vi "ConfigToIni.vi"(8 "Error In":errorcluster[](array[cluster]), 11 "ConfigRef":refnum<class "Config.lvclass">) -> (0 "Error Out":errorcluster[](array[cluster]), 3 "ConfigRef":refnum<class "Config.lvclass">)   [LabVIEW 2014, in "Config_class.lvlib" / "Config.lvclass"]
uses:
  Config.lvclass
  Typedefs/eLogLvl.ctl
  Config.lvclass/Config.ctl
  Accessors/Read ConfigFilePath.vi
  Accessors/Read Logging.vi
  Accessors/Read Root Directory.vi
  <vilib>/Utility/config.llb/NI_LVConfig.lvlib
  <userlib>/NIST/NISTErrorLib/NISTErrorLib.lvlib
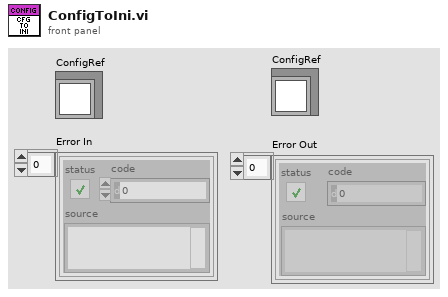
[diagram p1: front panel]
types:
  T1 = cluster{"pathRootDir":path, "OutDir":string, "ScriptDir":string, "TestDir":string}
  T2 = typedef "Config_class.lvlib/Config.lvclass/eLogLvl.ctl" = enum16{"Normal", "Verbose", "None"}
  T3 = typedef "Framework.lvlib/Config.lvclass/Logging.ctl" = cluster{"eLogLvl":T4, "Log File Path":path, "btnLogFile":bool}
  T4 = typedef "Framework.lvlib/Config.lvclass/eLogLvl.ctl" = enum16{"Normal", "Verbose", "None"}
  T5 = typedef "Config_class.lvlib/Config.lvclass/RootDir.ctl" = cluster{"pathRootDir":path, "btnOutPath":bool, "OutDir":string, "btnOpenOutputDir":bool, "ScriptDir":string, "btnOpenScriptDir":bool, "TestDir":string, "btnOpenTestDir":bool}
  T6 = typedef "NI_LVConfig.lvlib/Config Data RefNum.ctl" = refnum<k1>
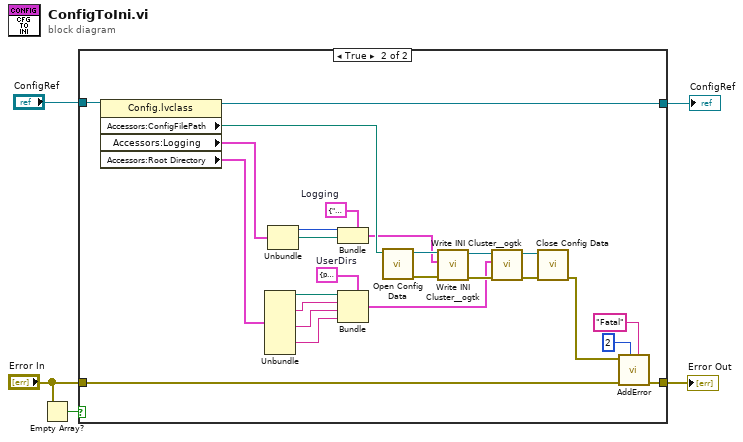
[diagram p0: block diagram]
diagram:
  n1 = Empty Array?(array="Error In") -> (empty?=w3:bool)
  n2 = case shown="True" w3 {
    tunnel: "ConfigRef" -> [w6 w33]
    tunnel: [w6 w15] -> w4
    tunnel: "Error In" -> [w7 w14]
    tunnel: [w7 w11] -> w1
    frame False {
    }
    frame True {
      w8 = T1 {"pathRootDir"=path "", "OutDir"="", "ScriptDir"="", "TestDir"=""}  # UserDirs
      w9 = cluster{"eLogLvl":T2, "Log File Path":path} {"eLogLvl"=enum."Normal", "Log File Path"=path ""}  # Logging
      n3 = property class="Config.lvclass"(reference=w33) -> (reference out=w15:refnum<class "Config.lvclass">, "Accessors:ConfigFilePath"=w21:path, "Accessors:Logging"=w28:T3, "Accessors:Root Directory"=w27:T5)  [unwired: 1 in, 1 out]
      n4 = Unbundle(w27) -> ("pathRootDir"=w32:path, "OutDir"=w31:string, "ScriptDir"=w30:string, "TestDir"=w29:string)  [unwired: 4 out]
      n5 = Unbundle(w28) -> ("eLogLvl"=w26:T4, "Log File Path"=w25:path)  [unwired: 1 out]
      n6 = Bundle(cluster=w9, "eLogLvl"=w26, "Log File Path"=w25) -> (w17:cluster{"eLogLvl":T2, "Log File Path":path})
      n7 = Bundle(cluster=w8, "pathRootDir"=w32, "OutDir"=w31, "ScriptDir"=w30, "TestDir"=w29) -> (w16:T1)
      n8 = call <vilib>:"Open Config Data.vi"("configuration file path"=w21) -> ("error out"=w22:errorcluster, "refnum"=w20:T6)  [unwired: 8 in, 1 out]
      n9 = call <userlib>:"Write INI Cluster__ogtk.vi"("error in (no error)"=w22, "INI Fomatted Cluster"=w17, "refnum"=w20) -> ("error out"=w23:errorcluster, "dup refnum"=w19:T6)  [unwired: 7 in]
      n10 = call <userlib>:"Write INI Cluster__ogtk.vi"("error in (no error)"=w23, "INI Fomatted Cluster"=w16, "refnum"=w19) -> ("error out"=w24:errorcluster, "dup refnum"=w18:T6)  [unwired: 7 in]
      n11 = call <vilib>:"Close Config Data.vi"("error in (no error)"=w24, "refnum"=w18) -> ("error out"=w10:errorcluster)  [unwired: 8 in, 1 out]
      n12 = call <userlib>:"AddError.vi"("Severity"="Fatal", "Priority"=u8 2, "ErrorArray"=w14, "error in (no error)"=w10) -> ("ErrorArray"=w11:errorcluster[])  [unwired: 6 in, 1 out]
    }
  }
  "ConfigRef" <- w4
  "Error Out" <- w1
